vi "ERROR_HANDLE_TEST.vi"() -> ()   [LabVIEW 2025]
uses:
  STM-Auto-Project/QMH CTLS/Sweeper.ctl
panel:
  in  "error in (no error)":errorcluster={"status"=FALSE, "code"=0, "source"="Test"}
  out "error out":errorcluster
  out "remaining elements 2":T1[](array[typedef])
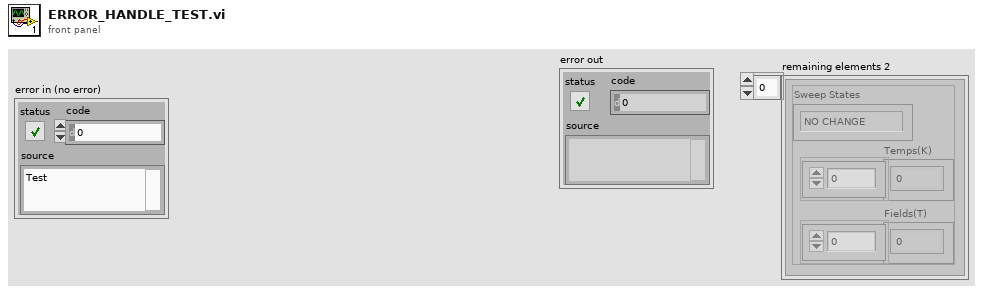
[diagram p1: front panel]
types:
  T1 = typedef "Sweeper.ctl" = cluster{"Temps(K)":dbl[], "Fields(T)":dbl[], "Sweep States":enum16{"NO CHANGE", "SET TEMP & FIELD", "SWEEP IDLE", "NEXT TEMP & FIELD", "SWEEP DONE"}}
  T2 = enum16{"NO CHANGE", "SET TEMP & FIELD", "SWEEP IDLE", "NEXT TEMP & FIELD", "SWEEP DONE"}
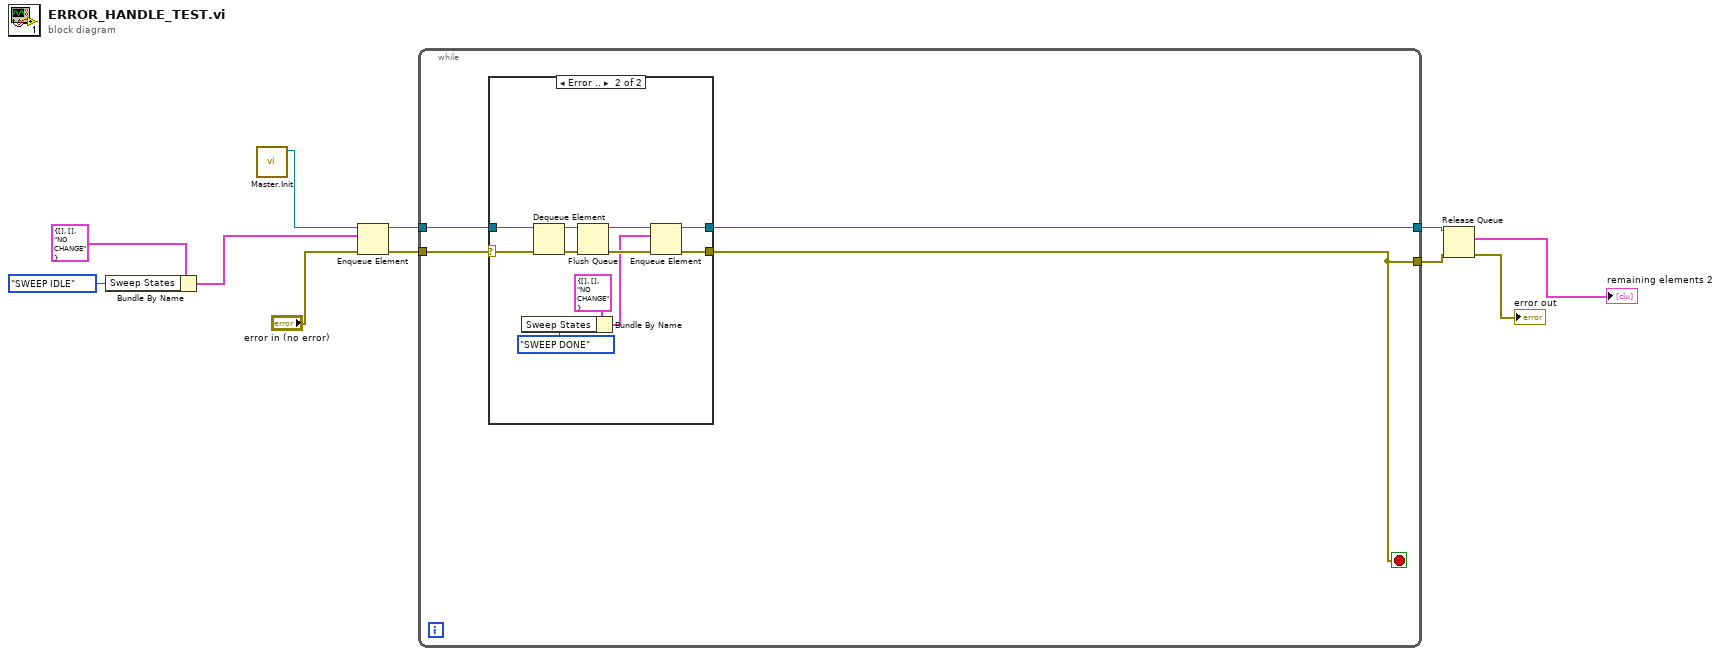
[diagram p0: block diagram]
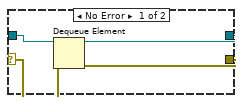
[diagram p2: hidden frame]
diagram:
  n1 = Bundle By Name(cluster=T1 {"Temps(K)"=[], "Fields(T)"=[], "Sweep States"=enum."NO CHANGE"} ("element"), "Sweep States"=T2."SWEEP IDLE") -> (w8:T1)
  n2 = call "Master.Init.vi"() -> ("SweepQ"=w11:refnum<queue>)  [unwired: 8 in, 3 out]
  n3 = Enqueue Element(queue=w11, element=w8, error in (no error)="error in (no error)") -> (queue out=w7:refnum<queue>, error out=w5:errorcluster)  [unwired: 1 in, 1 out]
  n4 = while {
    tunnel: w7 -> [w15]
    tunnel: w5 -> [w14]
    tunnel: [w13] -> w3
    tunnel: [w12] -> w4
    stop <- w12 stop-if-true
    n5 = case shown="Error .." w14 {
      selector: w14 -> [w19 w30]
      tunnel: w15 -> [w18 w29]
      tunnel: [w17 w21] -> w13
      tunnel: [w16 w20] -> w12
      frame No Error {
        n6 = Dequeue Element(queue=w18, error in (no error)=w19) -> (queue out=w17:refnum<queue>, error out=w16:errorcluster)  [unwired: 1 in, 2 out]
      }
      frame Error {
        n7 = Bundle By Name(cluster=T1 {"Temps(K)"=[], "Fields(T)"=[], "Sweep States"=enum."NO CHANGE"} ("element"), "Sweep States"=T2."SWEEP DONE") -> (w22:T1)
        n8 = Dequeue Element(queue=w29, error in (no error)=w30) -> (queue out=w27:refnum<queue>, error out=w28:errorcluster)  [unwired: 1 in, 2 out]
        n9 = Flush Queue(queue=w27, error in (no error)=w28) -> (queue out=w25:refnum<queue>, error out=w26:errorcluster)  [unwired: 1 out]
        n10 = Enqueue Element(queue=w25, element=w22, error in (no error)=w26) -> (queue out=w21:refnum<queue>, error out=w20:errorcluster)  [unwired: 1 in, 1 out]
      }
    }
  }
  n11 = Release Queue(queue=w3, error in (no error)=w4) -> (remaining elements=→"remaining elements 2":T1[], error out=→"error out":errorcluster)  [unwired: 1 in, 1 out]
